vi "Go To Assessing.vi"(8 "error in (no error)":errorcluster, 11 "EL-Go To Height in":refnum<class "EL-Go To Height.lvclass">) -> (0 "error out":errorcluster, 3 "State out":refnum<class "State Actor.lvclass">)   [LabVIEW 2014, in "Elevator.lvlib" / "EL-Go To Height.lvlib" / "EL-Go To Height.lvclass"]
uses:
  EL-Go To Height.lvclass
  <vilib>/ni/Actors/State Actor/State Actor/State Actor.lvclass
  GTH-Assessing Class/GTH-Assessing.lvclass
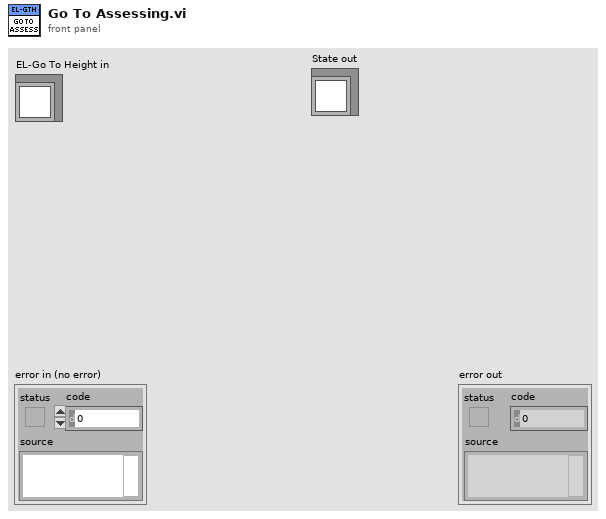
[diagram p1: front panel]
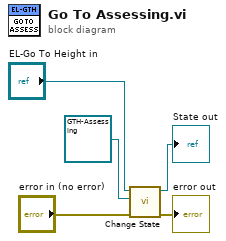
[diagram p0: block diagram]
diagram:
  n1 = call <vilib>:"Change State.vi"("error in (no error)"="error in (no error)", "New State in"=refnum<class "GTH-Assessing.lvclass"> refnum ("Elevator.lvlib:EL-Go To Height.lvlib:GTH-Assessing.lvclass"), "State in"="EL-Go To Height in") -> ("error out"=→"error out":errorcluster, "State out"=→"State out":refnum<class "State Actor.lvclass">)  [unwired: 7 in]
